vi "Get All VI Data.vi"(8 "error in (no error)":errorcluster, 10 "Abbreviate Names?":bool, 11 "All Files in Dir":path[](array[path])) -> (0 "error out":errorcluster, 2 "Names":string[](array[string]), 3 "VI Data":T1[](array[typedef]))   [LabVIEW 2023, in "VI Properties Editor.lvlib"]
uses:
  VI Properties Editor.lvlib
  Cluster Data.ctl
  <vilib>/picture/picture.llb/imagedata.ctl
  VI Properties.ctl
  Control Properties.ctl
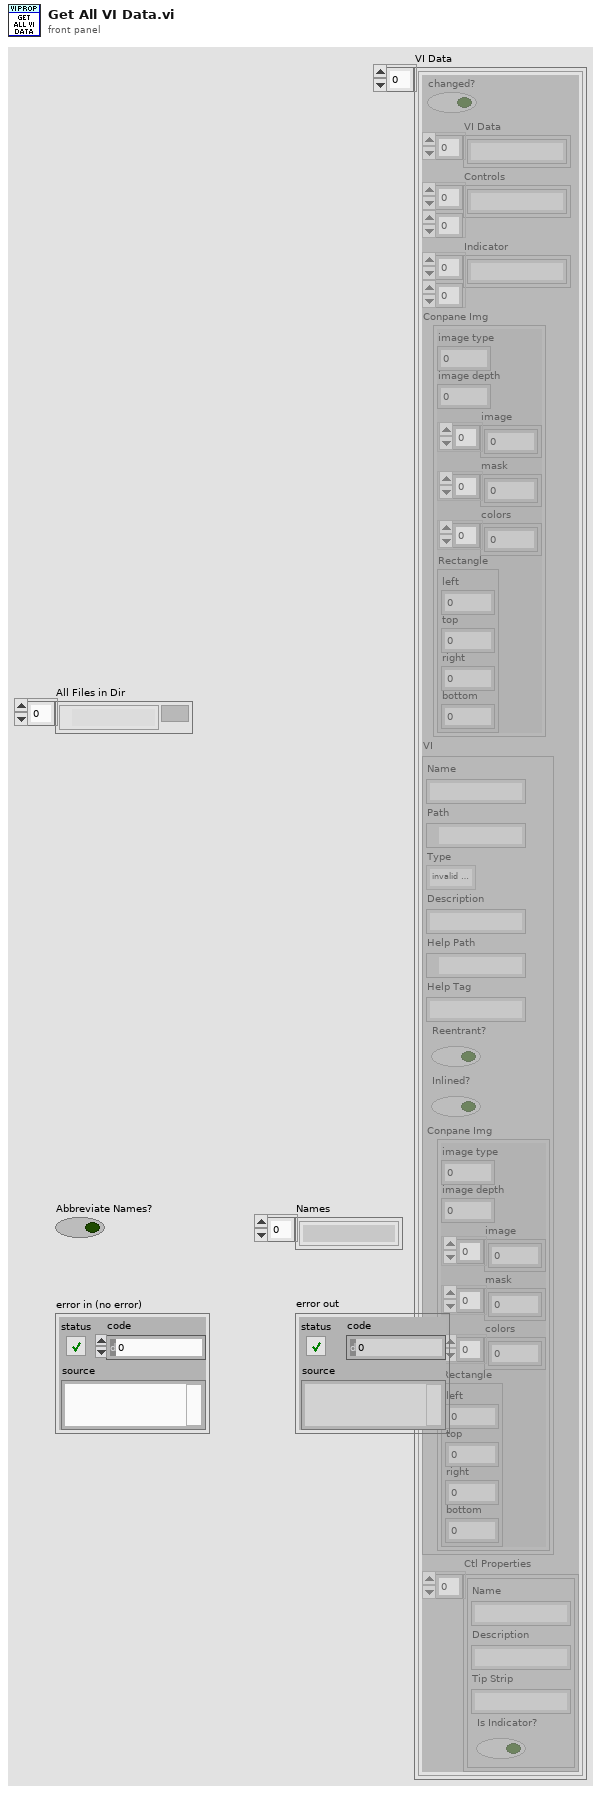
[diagram p1: front panel]
types:
  T1 = typedef "VI Properties Editor.lvlib/Cluster Data.ctl" = cluster{"changed?":bool, "VI Data":string[], "Controls":string[][], "Indicator":string[][], "Conpane Img":T2, "VI":T3, "Ctl Properties":T4[]}
  T2 = typedef "imagedata.ctl" = cluster{"image type":i32, "image depth":i32, "image":u8[], "mask":u8[], "colors":u32[], "Rectangle":cluster{"left":i16, "top":i16, "right":i16, "bottom":i16}}
  T3 = typedef "VI Properties Editor.lvlib/VI Properties.ctl" = cluster{"Name":string, "Path":path, "Type":enum32{"invalid VI type", "Standard VI", "Control VI", "Global VI", "Polymorphic VI", "Configuration VI", "SubSystem", "Facade VI", "Method VI", "Statechart Diagram VI"}, "Description":string, "Help Path":path, "Help Tag":string, "Reentrant?":bool, "Inlined?":bool, "Conpane Img":T2}
  T4 = typedef "VI Properties Editor.lvlib/Control Properties.ctl" = cluster{"Name":string, "Description":string, "Tip Strip":string, "Is Indicator?":bool}
  T5 = enum32{"invalid VI type", "Standard VI", "Control VI", "Global VI", "Polymorphic VI", "Configuration VI", "SubSystem", "Facade VI", "Method VI", "Statechart Diagram VI"}
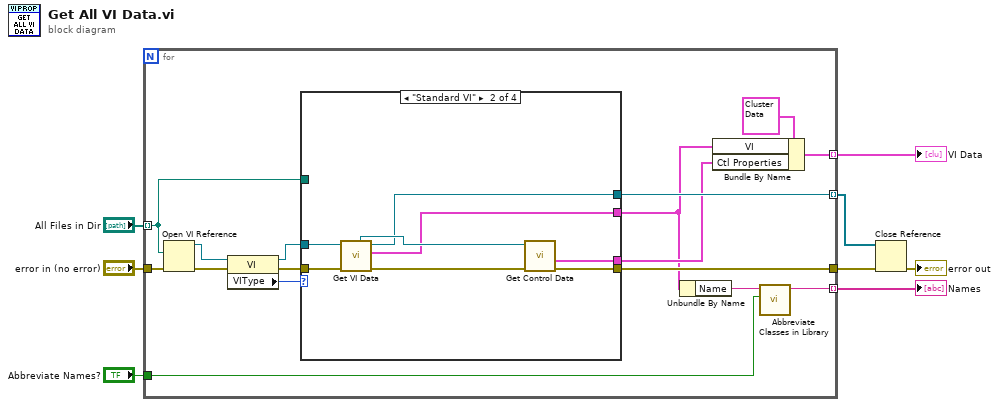
[diagram p0: block diagram]
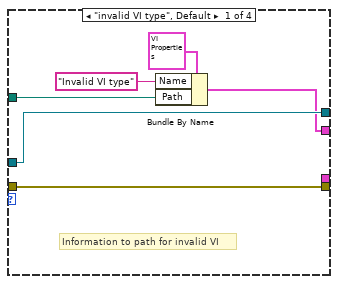
[diagram p2: hidden frame]
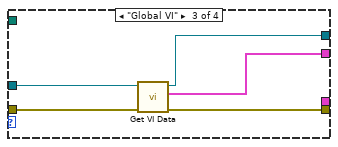
[diagram p3: hidden frame]
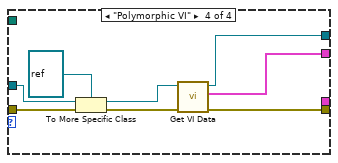
[diagram p4: hidden frame]
diagram:
  n1 = for {
    tunnel: "error in (no error)" -> [w23]
    tunnel: "All Files in Dir" -> [w14] mode=indexing
    tunnel: [w16] -> w6 mode=indexing
    tunnel: [w19] -> w3
    tunnel: [w18] -> w2 mode=indexing
    tunnel: [w17] -> w4 mode=indexing
    tunnel: "Abbreviate Names?" -> [w13]
    n2 = Open VI Reference(vi path=w14, error in (no error)=w23) -> (vi reference=w15:refnum<vi>, error out=w24:errorcluster)  [unwired: 4 in]
    n3 = property class="VI"(reference=w15, error in=w24) -> (reference out=w21:refnum<vi>, error out=w22:errorcluster, "VIType"=w20:T5)
    n4 = case shown="\"Standard VI\"" w20 {
      tunnel: w22 -> [w30 w38 w43 w50]
      tunnel: w21 -> [w29 w37 w41 w49]
      tunnel: [w25 w32 w39 w44] -> w10
      tunnel: [w30 w33 w42 w46] -> w19
      tunnel: [w29 w34 w40 w45] -> w18
      tunnel: w14 -> [w26 _ _ _]
      tunnel: [_ w31 _ _] -> w11
      frame "invalid VI type", Default {
        # "Information to path for invalid VI"
        n5 = Bundle By Name(cluster=T3 {"Name"="", "Path"=path "", "Type"=enum."invalid VI type", "Description"="", "Help Path"=path "", "Help Tag"="", "Reentrant?"=FALSE, "Inlined?"=FALSE, "Conpane Img"={"image type"=0, "image depth"=0, "image"=[], "mask"=[], "colors"=[], "Rectangle"={"left"=0, "top"=0, "right"=0, "bottom"=0}}} ("VI Properties"), "Name"="Invalid VI type" ("Help.Tag"), "Path"=w26) -> (w25:T3)
      }
      frame "Standard VI" {
        n6 = call "Get VI Data.vi"("error in (no error)"=w38, "VI in"=w37) -> ("error out"=w36:errorcluster, "VI Properties"=w32:T3, "VI out"=w34:refnum<vi>, "Panel"=w35:refnum<vi>)  [unwired: 6 in]
        n7 = call "Get Control Data.vi"("error in (no error)"=w36, "Panel"=w35) -> ("error out"=w33:errorcluster, "Control Data"=w31:T4[])  [unwired: 6 in, 2 out]
      }
      frame "Global VI" {
        n8 = call "Get VI Data.vi"("error in (no error)"=w43, "VI in"=w41) -> ("error out"=w42:errorcluster, "VI Properties"=w39:T3, "VI out"=w40:refnum<vi>)  [unwired: 6 in, 1 out]
      }
      frame "Polymorphic VI" {
        n9 = To More Specific Class(target class=refnum<vi> refnum, reference=w49, error in=w50) -> (specific class reference=w47:refnum<vi>, error out=w48:errorcluster)
        n10 = call "Get VI Data.vi"("error in (no error)"=w48, "VI in"=w47) -> ("error out"=w46:errorcluster, "VI Properties"=w44:T3, "VI out"=w45:refnum<vi>)  [unwired: 6 in, 1 out]
      }
    }
    n11 = Unbundle By Name(w10) -> ("Name"=w9:string)
    n12 = Bundle By Name(cluster=T1 {"changed?"=FALSE, "VI Data"=[], "Controls"=[], "Indicator"=[], "Conpane Img"={"image type"=0, "image depth"=0, "image"=[], "mask"=[], "colors"=[], "Rectangle"={"left"=0, "top"=0, "right"=0, "bottom"=0}}, "VI"={"Name"="", "Path"=path "", "Type"=enum."invalid VI type", "Description"="", "Help Path"=path "", "Help Tag"="", "Reentrant?"=FALSE, "Inlined?"=FALSE, "Conpane Img"={"image type"=0, "image depth"=0, "image"=[], "mask"=[], "colors"=[], "Rectangle"={"left"=0, "top"=0, "right"=0, "bottom"=0}}}, "Ctl Properties"=[]}, "VI"=w10, "Ctl Properties"=w11) -> (w17:T1)
    n13 = call "Abbreviate Classes in Library.vi"("Abbreviate Name?"=w13, "Name in"=w9) -> ("Name out"=w16:string)  [unwired: 9 in]
  }
  "Names" <- w6
  "VI Data" <- w4
  n14 = Close Reference(reference=w2, error in (no error)=w3) -> (error out=→"error out":errorcluster)
